vi "Configure Modulation (Frequency).vi"(0 "VISA resource name":refnum<visa-resource-name>, 1 "Enable FM (T:Enable)":bool=TRUE, 2 "FM Path (1)":u16(ring)=1 items=["1"=1, "2"=2], 5 "Enable Deviation Coupling (T:Enable)":bool=TRUE, 7 "FM Deviation (1000 Hz)":dbl=1000.0, 11 "error in (no error)":errorcluster) -> (4 "VISA resource name out":refnum<visa-resource-name>, 15 "error out":errorcluster)   [LabVIEW 2012, in "Agilent PSG MXG Series.lvlib"]
doc: "Configures frequency modulation.\n\n<B>Notes:</B>\n(1) This VI is <B>NOT</B> valid in E8247C.\n\n(2) For E8257D, E8267D, N5161A, N5162A, N5181A, N5182A, N5183A, N5171B, N5172B, N5181B, N5182B, this VI is valid only when the instument installs <B>Option UNT</B> (AM, FM, phase modulation)."
uses:
  <instrlib>/Agilent PSG MXG Series/Agilent PSG MXG Series.lvlib
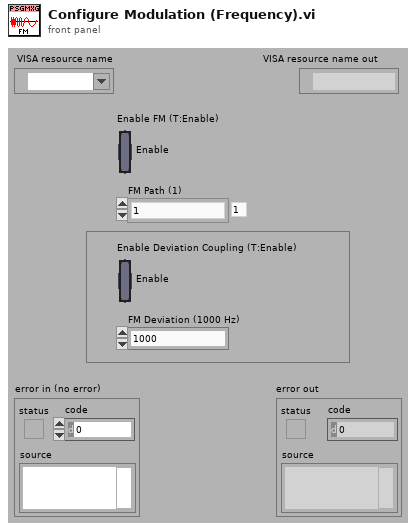
[diagram p1: front panel]
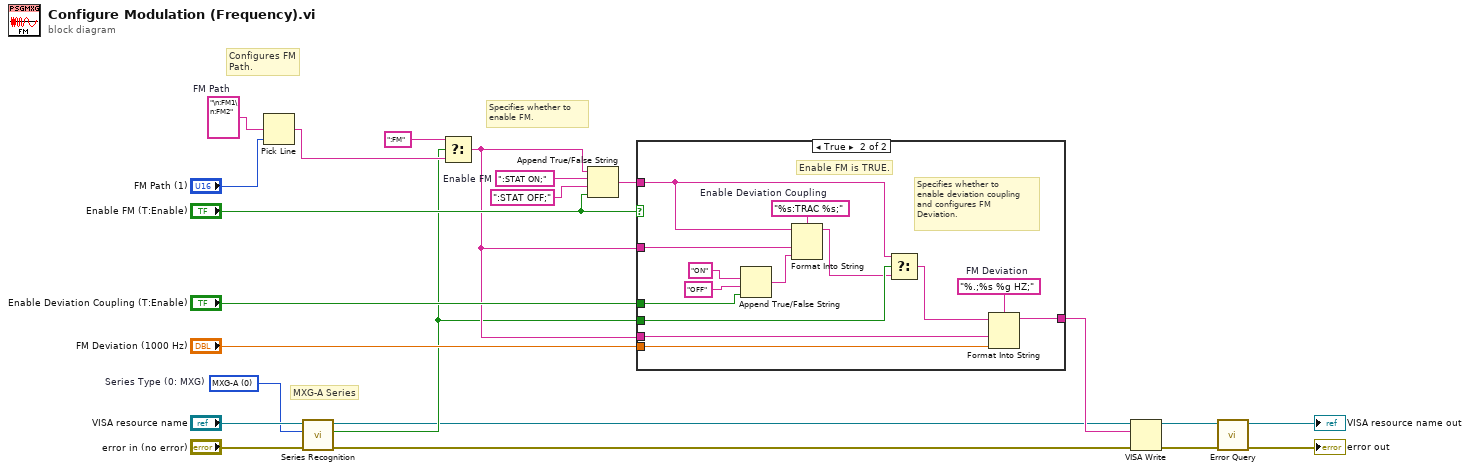
[diagram p0: block diagram]
diagram:
  w1 = u16 0 items=["MXG-A", "PSG", "PSG-A", "PSG-C", "PSG-D", "MXG-B", "EXG"]  # Series Type (0: MXG)
  w18 = ":STAT ON;"  # Enable FM
  w22 = "\n:FM1\n:FM2"  # FM Path
  # "MXG-A Series"
  # "Configures FM\nPath."
  # "Specifies whether to\nenable FM."
  n1 = Pick Line(multi-line string=w22, line index="FM Path (1)") -> (output string=w20:string)  [unwired: 1 out]
  n2 = call <instrlib>:"Series Recognition.vi"("error in (no error)"="error in (no error)", "Series Type (0: MXG)"=w1, "VISA resource name"="VISA resource name") -> ("error out"=w6:errorcluster, "Is Series Correct"=w8:bool, "VISA resource name out"=w7:refnum<visa-resource-name>)  [unwired: 6 out]
  n3 = Select(t=":FM", s=w8, f=w20) -> (s? t:f=w11:string)
  n4 = Append True/False String(1:"Enable FM (T:Enable)", 2:":STAT OFF;" ("true string"), 3:w18, 4:w11) -> (0:w12:string)
  n5 = case shown="True" "Enable FM (T:Enable)" {
    tunnel: w11 -> [_ w36]
    tunnel: "Enable Deviation Coupling (T:Enable)" -> [_ w33]
    tunnel: w8 -> [_ w32]
    tunnel: w12 -> [w23 w31]
    tunnel: w11 -> [_ w27]
    tunnel: "FM Deviation (1000 Hz)" -> [_ w26]
    tunnel: [w23 w25] -> w9
    frame False {
      # "Enable FM is FALSE."
    }
    frame True {
      w29 = "%.;%s %g HZ;"  # FM Deviation
      w37 = "%s:TRAC %s;"  # Enable Deviation Coupling
      # "Specifies whether to\nenable deviation coupling\nand configures FM\nDeviation."
      # "Enable FM is TRUE."
      n6 = Append True/False String(1:w33, 2:"OFF" ("false string"), 3:"ON" ("true string")) -> (0:w35:string)  [unwired: 1 out]
      n7 = Format Into String(format string=w37, initial string=w31, w36, w35) -> (resulting string=w30:string)  [unwired: 1 in, 1 out]
      n8 = Select(t=w31, s=w32, f=w30) -> (s? t:f=w28:string)
      n9 = Format Into String(format string=w29, initial string=w28, w27, w26) -> (resulting string=w25:string)  [unwired: 1 in, 1 out]
    }
  }
  n10 = VISA Write(VISA resource name=w7, write buffer=w9, error in (no error)=w6) -> (VISA resource name out=w15:refnum<visa-resource-name>, error out=w14:errorcluster)  [unwired: 1 out]
  n11 = call <instrlib>:"Error Query.vi"("error in (no error)"=w14, "VISA resource name"=w15) -> ("error out"=→"error out":errorcluster, "VISA resource name out"=→"VISA resource name out":refnum<visa-resource-name>)  [unwired: 8 out]
